vi "Vision Research Phantom Series PhCon PhPhGetCineCount.vi"(0 "CN in":u32=1, 5 "Error In (no error)":errorcluster) -> (14 "CN out":u32=1, 16 "pRAMCount":u32, 17 "pNVMCount":u32, 19 "Error Out":errorcluster)   [LabVIEW 2013, in "VRI.lvlib"]
doc: "PhCon.dll\n\nPhGetCineCount\nHRESULT PhGetCineCount(UINT CN, PUINT pRAMCount, PUINT pNVMCount);\n\nParameters Description\nCN(in) Camera Number.\npRAMCount(out) The number of cines stored in the camera RAM. Can be more \n than 1 if the camera supports the multi-cine.\npNVMCount(out) The numbers of cines stored in the camera NVM. To access \n these cines, use values starting at FIRST_FLASH_CINE.\nReturn (0 = Ok)\nComments Counts the cines available for playback from the camera, \n both in RAM and in NVM."
uses:
  VRI.lvlib
  Phantom DLLs/PhCon.dll
panel:
  # "For instructions on the use of this VI, press Ctrl+H to display the help window and move the mouse over the icon, controls, and indicators"
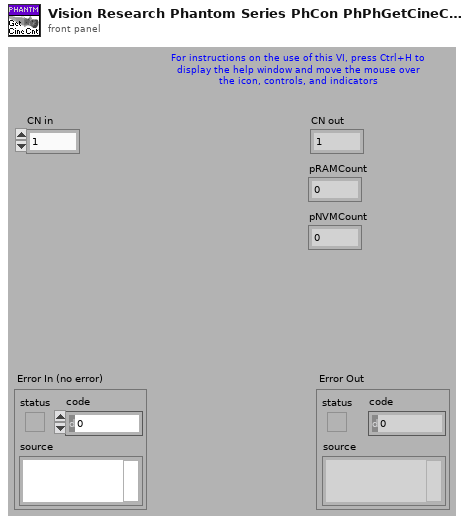
[diagram p1: front panel]
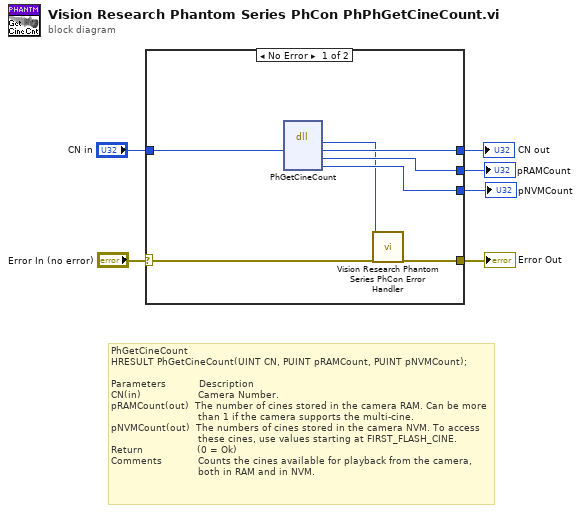
[diagram p0: block diagram]
diagram:
  # "PhGetCineCount\nHRESULT PhGetCineCount(UINT CN, PUINT pRAMCount, PUINT pNVMCount);\n\nParameters           Description\nCN(in)                   Camera Number.\npRAMCount(out)  The number of cines stored in the camera RAM. Can be more \n                             than 1 if the camera supports the multi-cine.\npNVMCount(out)  The numbers of cines stored in the camera NVM. To access  \n                             these cines, use values starting at FIRST_FLASH_CINE.\nReturn                  (0 = Ok)\nComments            Counts the cines available for playback from the camera, \n                             both in RAM and in NVM."
  n1 = case shown="No Error" "Error In (no error)" {
    selector: "Error In (no error)" -> [w13 w15]
    tunnel: [w12 w15] -> w5
    tunnel: "CN in" -> [w11 w14]
    tunnel: [w10 w14] -> w3
    tunnel: [w9 _] -> w2
    tunnel: [w8 _] -> w1
    frame No Error {
      n2 = dll-call lib="C:/Projects/SDK/32-bit/Vision Research Phantom Series Labview Driver/Phantom DLLs/PhCon.dll" fn="PhGetCineCount"("CN"=w11) -> ("HRESULT"=w7:i32, "CN"=w10:u32, "pRamCount"=w9:u32, "pNVMCount"=w8:u32)  [unwired: 3 in, 4 out]
      n3 = call "Vision Research Phantom Series PhCon Error Handler.vi"("ErrNo"=w7, "Error In (no error)"=w13) -> ("Error Out"=w12:errorcluster)  [unwired: 17 out]
    }
    frame Error {
    }
  }
  "Error Out" <- w5
  "CN out" <- w3
  "pRAMCount" <- w2
  "pNVMCount" <- w1
